vi "AutoSingleDOF.vi"(0 "Auto Heading":bool, 1 "PID gains head":T1, 2 "SET MANUAL":bool, 3 "output range":cluster{"output high":dbl, "output low":dbl}, 5 "Integrator Reset":bool, 7 "varNumber":i32, 9 "Sampling Time":dbl, 11 "States":T2, 12 "Boolean":bool, 13 "delta REF":dbl, 14 "Numeric":dbl) -> (4 "set point":dbl, 6 "auto set":bool, 10 "output":dbl)   [LabVIEW 2014, in "Controller Library.lvlib" / "Oculus Rift Controller.lvclass"]
uses:
  Oculus Rift Controller.lvclass
  <vilib>/addons/control/pid/pid.llb/PID (DBL).vi
  <vilib>/addons/control/pid/NI_PID_pid.lvlib
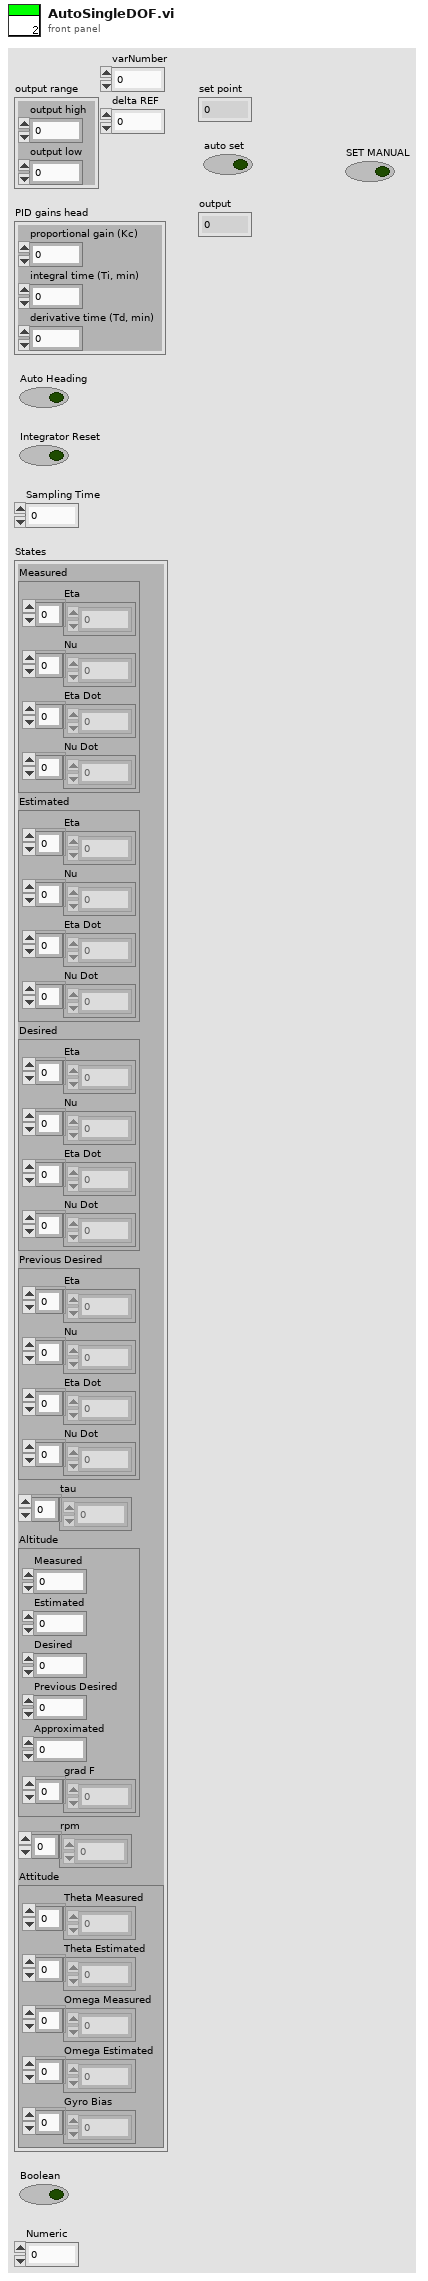
[diagram p1: front panel]
types:
  T1 = cluster{"proportional gain (Kc)":dbl, "integral time (Ti, min)":dbl, "derivative time (Td, min)":dbl}
  T2 = cluster{"Measured":cluster{"Eta":dbl[], "Nu":dbl[], "Eta Dot":dbl[], "Nu Dot":dbl[]}, "Estimated":cluster{"Eta":dbl[], "Nu":dbl[], "Eta Dot":dbl[], "Nu Dot":dbl[]}, "Desired":cluster{"Eta":dbl[], "Nu":dbl[], "Eta Dot":dbl[], "Nu Dot":dbl[]}, "Previous Desired":cluster{"Eta":dbl[], "Nu":dbl[], "Eta Dot":dbl[], "Nu Dot":dbl[]}, "tau":dbl[], "Altitude":cluster{"Measured":dbl, "Estimated":dbl, "Desired":dbl, "Previous Desired":dbl, "Approximated":dbl, "grad F":dbl[]}, "rpm":dbl[], "Attitude":cluster{"Theta Measured":dbl[], "Theta Estimated":dbl[], "Omega Measured":dbl[], "Omega Estimated":dbl[], "Gyro Bias":dbl[]}}
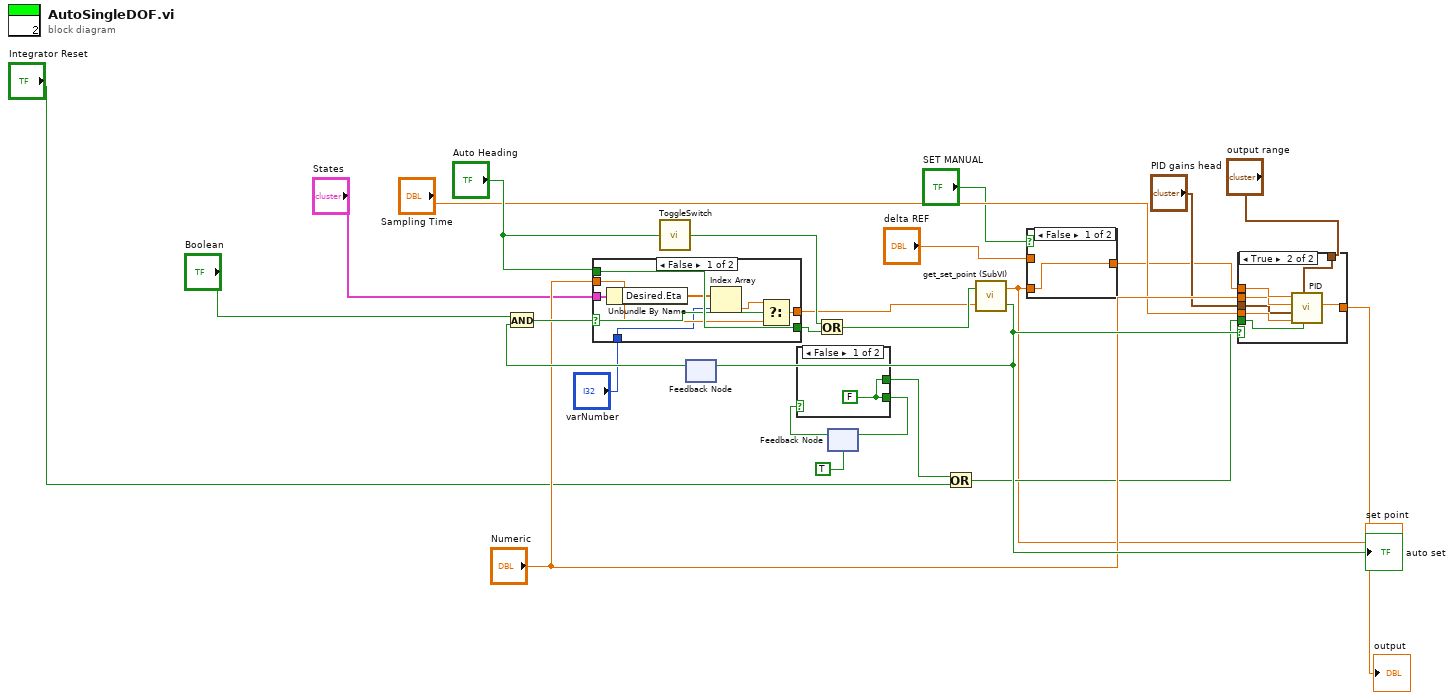
[diagram p0: block diagram]
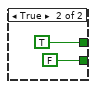
[diagram p3: hidden frame]
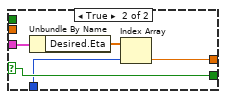
[diagram p4: hidden frame]
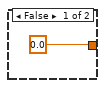
[diagram p5: hidden frame]
diagram:
  n1 = call "ToggleSwitch.vi"("Input"="Auto Heading") -> ("Output"=w21:bool)
  n2 = feedback #1() -> (w25:bool)  [unwired: 1 in]
  n3 = And(x="Boolean", y=w25) -> (x .and. y?=w24:bool)
  n4 = case shown="False" w24 {
    selector: w24 -> [w33 w36]
    tunnel: "States" -> [w31 w39]
    tunnel: [w32 w37] -> w7
    tunnel: "Numeric" -> [w28 _]
    tunnel: "Auto Heading" -> [w34 _]
    tunnel: [w34 w36] -> w8
    tunnel: "varNumber" -> [w27 w35]
    frame False {
      n5 = Unbundle By Name(w31) -> ("Desired.Eta"=w30:dbl[])
      n6 = Index Array(array=w30, index=w27) -> (element=w29:dbl)
      n7 = Select(t=w29, s=w33, f=w28) -> (s? t:f=w32:dbl)
    }
    frame True {
      n8 = Unbundle By Name(w39) -> ("Desired.Eta"=w38:dbl[])
      n9 = Index Array(array=w38, index=w35) -> (element=w37:dbl)
    }
  }
  n10 = Or(x=w21, y=w8) -> (x .or. y?=w9:bool)
  n11 = feedback #2(TRUE) -> (w18:bool)
  n12 = case shown="False" w18 {
    tunnel: [w40 FALSE] -> w19
    tunnel: [w40 TRUE] -> w22
    frame False {
      w40 = FALSE
    }
    frame True {
    }
  }
  n13 = feedback-in #2(w19) -> ()
  n14 = Or(x=w22, y="Integrator Reset") -> (x .or. y?=w12:bool)
  n15 = call "get_set_point (SubVI).vi"("set point in"=w7, "auto set  in"=w9) -> ("auto set"=w26:bool, "set point"=w4:dbl)
  "auto set" <- w26
  "set point" <- w4
  n16 = feedback-in #1(w26) -> ()
  n17 = case shown="False" "SET MANUAL" {
    tunnel: w4 -> [w43 _]
    tunnel: [w43 w44] -> w3
    tunnel: "delta REF" -> [_ w44]
    frame False {
    }
    frame True {
    }
  }
  n18 = case shown="True" w26 {
    tunnel: "output range" -> [_ w52]
    tunnel: "Sampling Time" -> [_ w51]
    tunnel: [0.0 ("output") w50] -> w16
    tunnel: w3 -> [_ w49]
    tunnel: "Numeric" -> [_ w48]
    tunnel: w12 -> [_ w47]
    tunnel: "PID gains head" -> [_ w46]
    frame False {
    }
    frame True {
      n19 = call-poly <vilib>:"PID.vi"("reinitialize? (F)"=w47, "output range"=w52, "dt (s)"=w51, "PID gains"=w46, "process variable"=w48, "setpoint"=w49) -> ("output"=w50:dbl)  [unwired: 4 in, 1 out]
    }
  }
  "output" <- w16
